vi "SetKeithleyAndStabilizeCell_Martina_Aging.vi"(2 "Liv/Div":bool, 3 "Scan Parameters":T1={"Scan Direction\nDU (T), UD (F)"=FALSE, "Maximum Voltage (V)"=2.0, "Minimum Voltage (V)"=1.0, "Stabilization Time (s)"=10.0, "Range Options"=0} {"Range Options" items=["Auto Range", "Semi-Auto Range", "100 uA", "1 mA", "10 mA", "100 mA", "1A"]}) -> (0 "error out":errorcluster, 1 "VISA resource name out":refnum<visa-resource-name>)   [LabVIEW 2011]
uses:
  C:/Program Files (x86)/National Instruments/LabVIEW 2009/instr.lib/Keithley 24XX/Keithley 24XX.lvlib
  C:/Program Files (x86)/National Instruments/LabVIEW 2009/instr.lib/Keithley 24XX/Public/Data/Read (Single Point).vi
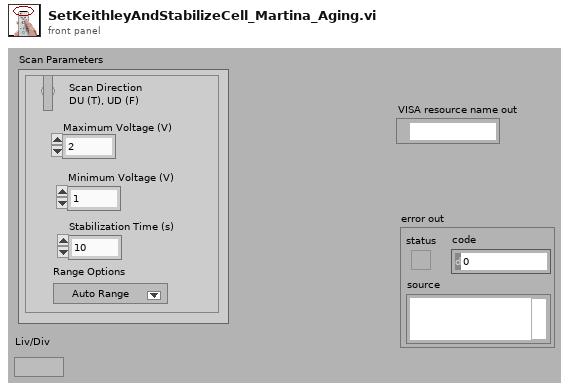
[diagram p1: front panel]
types:
  T1 = cluster{"Scan Direction\nDU (T), UD (F)":bool, "Maximum Voltage (V)":dbl, "Minimum Voltage (V)":dbl, "Stabilization Time (s)":dbl, "Range Options":u16}
  T2 = cluster{"Baud Rate":u32, "Parity":u16, "Data Bits":u16, "Stop Bits":u16, "Flow Control":u16}
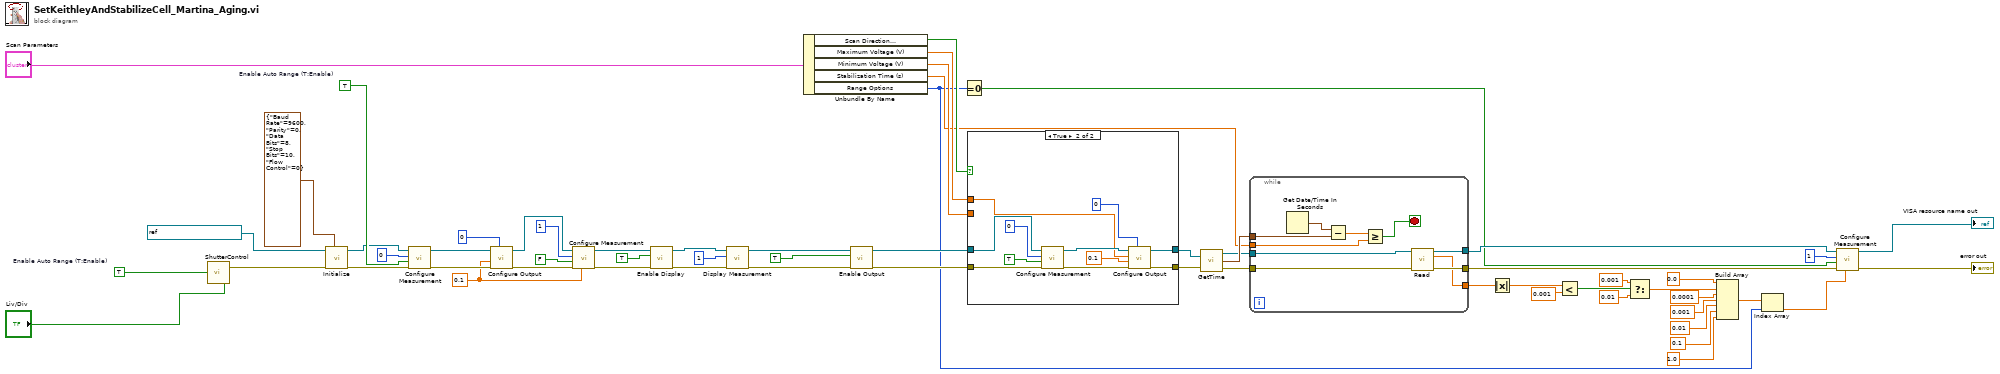
[diagram p0: block diagram]
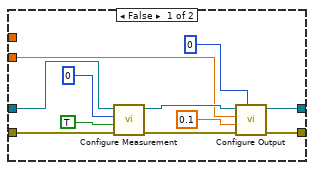
[diagram p2: hidden frame]
diagram:
  w26 = 0.1 ("Compliance  Level (0.1)")
  w37 = TRUE  # Enable Auto Range (T:Enable)
  w50 = TRUE  # Enable Auto Range (T:Enable)
  n1 = call "ShutterControl.vi"("Enable?"=w37, "ON/OFF"="Liv/Div") -> ("error out"=w38:errorcluster)
  n2 = call "Initialize.vi"("Serial Configuration"=T2 {"Baud Rate"=9600, "Parity"=0, "Data Bits"=8, "Stop Bits"=10, "Flow Control"=0}, "error in (no error)"=w38, "VISA resource name"=refnum<visa-resource-name> "KE2400ExampleInstr") -> ("error out"=w45:errorcluster, "VISA resource name out"=w44:refnum<visa-resource-name>)  [unwired: 2 in, 5 out]
  n3 = call "Configure Measurement.vi"("error in (no error)"=w45, "Enable Auto Range (T:Enable)"=w50, "Function (0: Volts)"=0, "VISA resource name"=w44) -> ("error out"=w46:errorcluster, "VISA resource name out"=w49:refnum<visa-resource-name>)  [unwired: 1 in, 5 out]
  n4 = call "Configure Output.vi"("Source Mode  (0: Voltage)"=0, "error in (no error)"=w46, "Compliance  Level (0.1)"=w26, "VISA resource name"=w49) -> ("error out"=w47:errorcluster, "VISA resource name out"=w48:refnum<visa-resource-name>)  [unwired: 2 in, 4 out]
  n5 = call "Configure Measurement.vi"("Manual Range (1.0)"=w26, "error in (no error)"=w47, "Enable Auto Range (T:Enable)"=FALSE, "Function (0: Volts)"=1, "VISA resource name"=w48) -> ("error out"=w42:errorcluster, "VISA resource name out"=w43:refnum<visa-resource-name>)  [unwired: 5 out]
  n6 = call "Enable Display.vi"("error in (no error)"=w42, "Enable Display (T: Enable)"=TRUE ("Enable Output (T: Enable)"), "VISA resource name"=w43) -> ("error out"=w54:errorcluster, "VISA resource name out"=w55:refnum<visa-resource-name>)  [unwired: 7 out]
  n7 = call "Display Measurement.vi"("error in (no error)"=w54, "Displayed Measurement (0: Voltage)"=1, "VISA resource name"=w55) -> ("error out"=w53:errorcluster, "VISA resource name out"=w56:refnum<visa-resource-name>)  [unwired: 7 out]
  n8 = Unbundle By Name("Scan Parameters") -> ("Scan Direction\nDU (T), UD (F)"=w5:bool, "Maximum Voltage (V)"=w4:dbl, "Minimum Voltage (V)"=w3:dbl, "Stabilization Time (s)"=w2:dbl, "Range Options"=w1:u16)
  n9 = call "Enable Output.vi"("error in (no error)"=w53, "Enable Output (T: Enable)"=TRUE, "VISA resource name"=w56) -> ("error out"=w39:errorcluster, "VISA resource name out"=w40:refnum<visa-resource-name>)  [unwired: 7 out]
  n10 = Equal To 0?(x=w1) -> (x = 0?=w17:bool)
  n11 = case shown="True" w5 {
    tunnel: w40 -> [w66 w78]
    tunnel: [w68 w76] -> w33
    tunnel: [w67 w75] -> w34
    tunnel: w39 -> [w65 w77]
    tunnel: w4 -> [_ w73]
    tunnel: w3 -> [w63 _]
    frame False {
      n12 = call "Configure Measurement.vi"("error in (no error)"=w65, "Enable Auto Range (T:Enable)"=TRUE, "Function (0: Volts)"=0, "VISA resource name"=w66) -> ("error out"=w70:errorcluster, "VISA resource name out"=w71:refnum<visa-resource-name>)  [unwired: 1 in, 5 out]
      n13 = call "Configure Output.vi"("Source Mode  (0: Voltage)"=0, "error in (no error)"=w70, "Compliance  Level (0.1)"=0.1, "Output Level (0)"=w63, "VISA resource name"=w71) -> ("error out"=w67:errorcluster, "VISA resource name out"=w68:refnum<visa-resource-name>)  [unwired: 1 in, 4 out]
    }
    frame True {
      n14 = call "Configure Measurement.vi"("error in (no error)"=w77, "Enable Auto Range (T:Enable)"=TRUE, "Function (0: Volts)"=0, "VISA resource name"=w78) -> ("error out"=w81:errorcluster, "VISA resource name out"=w82:refnum<visa-resource-name>)  [unwired: 1 in, 5 out]
      n15 = call "Configure Output.vi"("Source Mode  (0: Voltage)"=0, "error in (no error)"=w81, "Compliance  Level (0.1)"=0.1, "Output Level (0)"=w73, "VISA resource name"=w82) -> ("error out"=w75:errorcluster, "VISA resource name out"=w76:refnum<visa-resource-name>)  [unwired: 1 in, 4 out]
    }
  }
  n16 = call "GetTime.vi"("VISA resource name"=w33, "error in"=w34) -> ("VISA resource name out"=w31:refnum<visa-resource-name>, "current time"=w35:timestamp, "error out"=w32:errorcluster)
  n17 = while {
    tunnel: w31 -> [w92]
    tunnel: [w91] -> w24
    tunnel: w32 -> [w90]
    tunnel: [w89] -> w23
    tunnel: w2 -> [w88]
    tunnel: w35 -> [w85]
    tunnel: [w83] -> w19
    stop <- w87 stop-if-true
    n18 = Get Date/Time In Seconds() -> (seconds since 1Jan1904=w86:timestamp)
    n19 = Subtract(x=w86, y=w85) -> (x-y=w84:dbl)
    n20 = Greater Or Equal?(x=w84, y=w88) -> (x >= y?=w87:bool)
    n21 = call-poly "Read.vi"("VISA resource name"=w92, "error in (no error)"=w90) -> ("VISA resource name out"=w91:refnum<visa-resource-name>, "Current"=w83:sgl, "error out"=w89:errorcluster)  [unwired: 2 in, 9 out]
  }
  n22 = Absolute Value(x=w19) -> (abs(x)=w18:sgl)
  n23 = Less?(x=w18, y=0.001) -> (x < y?=w29:bool)
  n24 = Select(t=0.001, s=w29, f=0.01) -> (s? t:f=w16:dbl)
  n25 = Build Array(0.0 ("s? t:f"), w16, 0.0001 ("s? t:f"), 0.001 ("s? t:f"), 0.01 ("s? t:f"), 0.1 ("s? t:f"), 1.0 ("s? t:f")) -> (w9:dbl[])
  n26 = Index Array(array=w9, index=w1) -> (element=w8:dbl)
  n27 = call "Configure Measurement.vi"("Manual Range (1.0)"=w8, "error in (no error)"=w23, "Enable Auto Range (T:Enable)"=w17, "Function (0: Volts)"=1, "VISA resource name"=w24) -> ("error out"=→"error out":errorcluster, "VISA resource name out"=→"VISA resource name out":refnum<visa-resource-name>)  [unwired: 5 out]
